vi "GoBang_Prototype.vi"() -> ()   [LabVIEW 2013, in "GoBang.lvlib"]
uses:
  GoBang.lvlib
  typdefs/BoardField.ctl
  typdefs/GameState.ctl
panel:
  in  "OppColor":T1
  in  "Opponnents name":string
  in  "Color":T1
  in  "Your name":string
  out "Game over":bool
  out "Black won":bool
  out "White won":bool
  in  "State":T2
  in  "stone":T1
  in  "stop":bool
  out "GameBoard":T1[][](array[typedef])
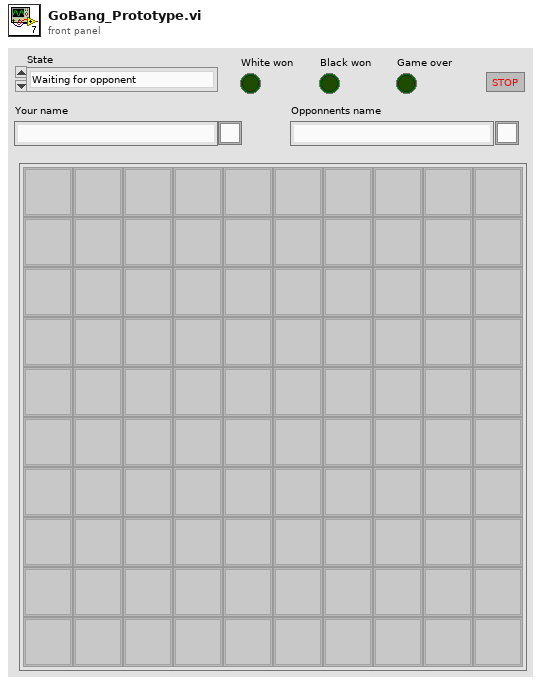
[diagram p1: front panel]
types:
  T1 = typedef "GoBang.lvlib/BoardField.ctl" = u8
  T2 = typedef "GoBang.lvlib/GameState.ctl" = enum16{"Waiting for opponent", "White to move", "Black to move", "Game over, white won", "Game over, black won"}
  T3 = typedef "LVPositionTypeDef.ctl" = cluster{"Left":i32, "Top":i32}
  T4 = typedef "LVBoundsTypeDef.ctl" = cluster{"Width":u32, "Height":u32}
  T5 = enum16{"Waiting for opponent", "White to move", "Black to move"}
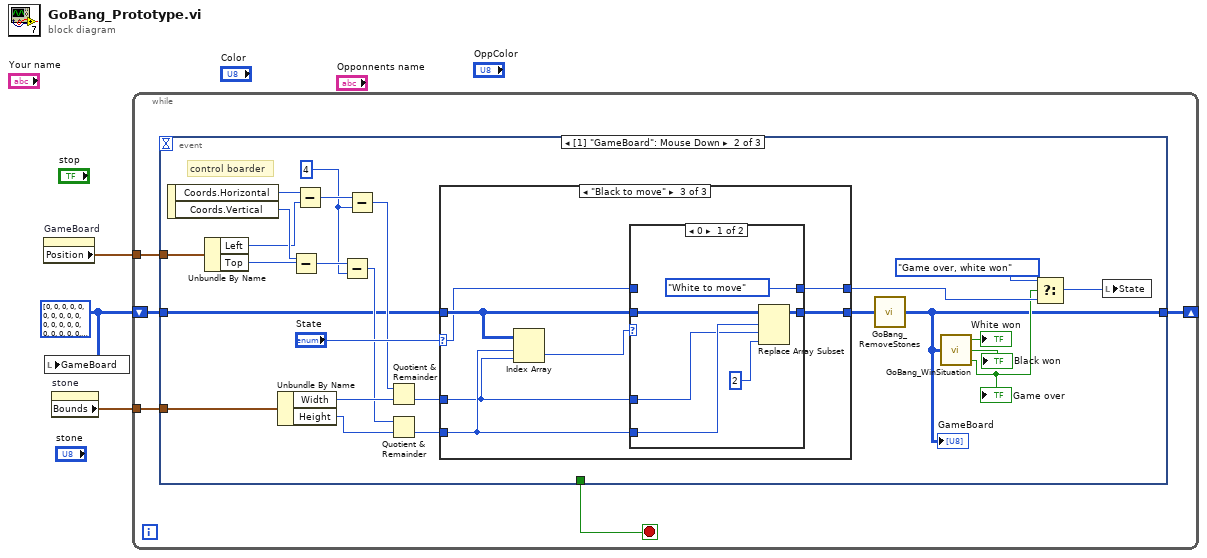
[diagram p0: block diagram]
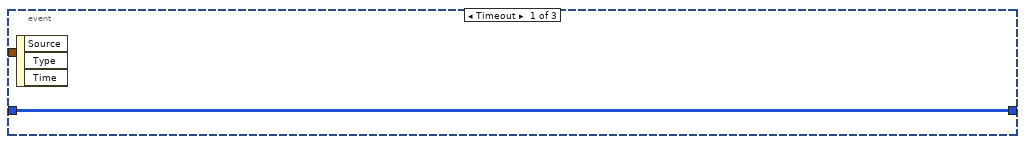
[diagram p2: hidden frame]
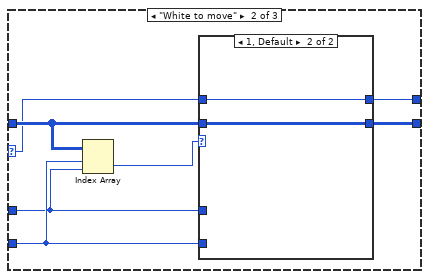
[diagram p4: hidden frame]
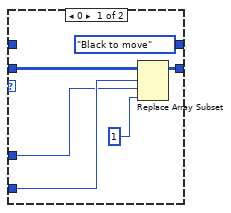
[diagram p5: hidden frame]
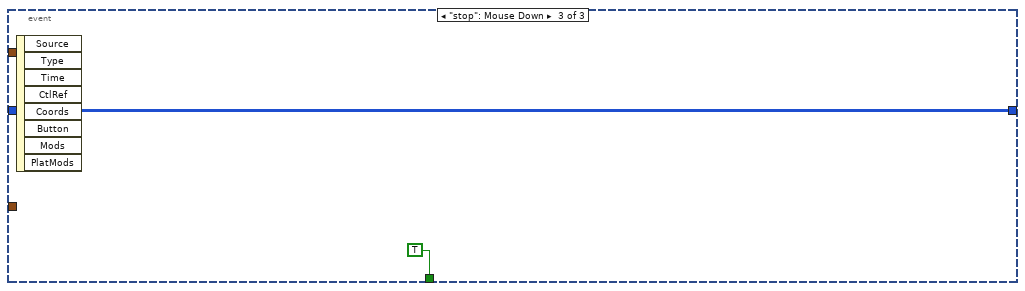
[diagram p7: hidden frame]
diagram:
  w1 = T1[][] [[0, 0, 0, 0, 0, 0, 0, 0, 0, 0], [0, 0, 0, 0, 0, 0, 0, 0, 0, 0], [0, 0, 0, 0, 0, 0, 0, 0, 0, 0], [0, 0, 0, 0, 0, 0, 0, 0, 0, 0], [0, 0, 0, 0, 0, 0, 0, 0, 0, 0], [0, 0, 0, 0, 0, 0, 0, 0, 0, 0], [0, 0, 0, 0, 0, 0, 0, 0, 0, 0], [0, 0, 0, 0, 0, 0, 0, 0, 0, 0], [0, 0, 0, 0, 0, 0, 0, 0, 0, 0], [0, 0, 0, 0, 0, 0, 0, 0, 0, 0]] ("GameBoard")
  n1 = property on="GameBoard" class="Arr (strict)"() -> ("Position"=w2:T3)  [unwired: 2 in, 2 out]
  n2 = local write "GameBoard"(w1) -> ()
  n3 = property on="stone" class="Ring (strict)"() -> ("Bounds"=w3:T4)  [unwired: 2 in, 2 out]
  n4 = while {
    tunnel: w3 -> [w7]
    tunnel: w2 -> [w6]
    shift-right: [w4] -> _
    shift-left: w1 -> [w5]
    stop <- w8 stop-if-true
    n5 = event shown="[1] \"GameBoard\": Mouse Down" {
      selector: _ -> [_ _ _]
      dyn-events: _ -> [_ _ _]
      timeout: _ -> [_ _ _]
      tunnel: [_ _ TRUE] -> w8
      tunnel: w7 -> [_ w33 _]
      tunnel: w6 -> [_ w28 _]
      tunnel: w5 -> [w9 w19 w67]
      tunnel: [w9 w10 w67] -> w4
      event Timeout {
        n6 = event-data() -> ()  [unwired: 1 in, 3 out]
      }
      event "GameBoard": Mouse Down {
        w21 = 4 ("y 2")
        # "control boarder"
        n7 = event-data() -> ("Coords.Horizontal"=w32:i32, "Coords.Vertical"=w30:i32)  [unwired: 1 in]
        n8 = Unbundle By Name(w28) -> ("Left"=w27:i32, "Top"=w26:i32)
        n9 = Unbundle By Name(w33) -> ("Width"=w31:u32, "Height"=w29:u32)
        n10 = Subtract(x=w30, y=w26) -> (x-y=w24:i32)
        n11 = Subtract(x=w32, y=w27) -> (x-y=w25:i32)
        n12 = Subtract(x=w24, y=w21) -> (x-y=w22:i32)
        n13 = Subtract(x=w25, y=w21) -> (x-y=w23:i32)
        n14 = Quotient & Remainder(x=w23, y=w31) -> (floor(x/y)=w18:u32)  [unwired: 1 out]
        n15 = Quotient & Remainder(x=w22, y=w29) -> (floor(x/y)=w17:u32)  [unwired: 1 out]
        n16 = case shown="\"Black to move\"" "State" {
          selector: "State" -> [w36 w37 w52]
          tunnel: [w36 w43 w58] -> w20
          tunnel: w19 -> [w35 w41 w56]
          tunnel: w18 -> [_ w39 w54]
          tunnel: w17 -> [_ w40 w55]
          tunnel: [w35 w42 w57] -> w11
          frame "Waiting for opponent", Default {
          }
          frame "White to move" {
            n17 = Index Array(array=w41, index (row)=w40, index (col)=w39) -> (element=w38:T1)
            n18 = case shown="1, Default" w38 {
              tunnel: [T5."Black to move" ("Mode") w51] -> w43
              tunnel: w41 -> [w48 w50]
              tunnel: [w46 w50] -> w42
              tunnel: w40 -> [w45 _]
              tunnel: w39 -> [w44 _]
              tunnel: w37 -> [_ w51]
              frame 0 {
                n19 = Replace Array Subset(array=w48, new element=T1 1 ("new element/subarray"), index (row)=w45, index (col)=w44) -> (w46:T1[][])
              }
              frame 1, Default {
              }
            }
          }
          frame "Black to move" {
            n20 = Index Array(array=w56, index (row)=w55, index (col)=w54) -> (element=w53:T1)
            n21 = case shown="0" w53 {
              tunnel: [GameState."White to move" ("State") w66] -> w58
              tunnel: w56 -> [w64 w65]
              tunnel: [w62 w65] -> w57
              tunnel: w55 -> [w61 _]
              tunnel: w54 -> [w60 _]
              tunnel: w52 -> [_ w66]
              frame 0 {
                n22 = Replace Array Subset(array=w64, new element=T1 2 ("new element/subarray"), index (row)=w61, index (col)=w60) -> (w62:T1[][])
              }
              frame 1, Default {
              }
            }
          }
        }
        n23 = call "GoBang_RemoveStones.vi"("GameBoard in"=w11) -> ("GameBoard out"=w10:u8[][])
        "GameBoard" <- w10
        n24 = call "GoBang_WinSituation.vi"("GameBoard"=w10) -> ("White won"=→"White won":bool, "Black won"=→"Black won":bool, "Game over"=w13:bool)
        "Game over" <- w13
        n25 = Select(t=GameState."Game over, white won" ("f"), s=w13, f=w20) -> (s? t:f=w14:T2)
        n26 = local write "State"(w14) -> ()
      }
      event "stop": Mouse Down {
        n27 = event-data() -> ()  [unwired: 1 in, 8 out]
      }
    }
  }
